vi "search for tag.vi"(8 "error in":errorcluster, 10 "system tag":refnum<class "tag descriptor.lvclass">, 11 "data dictionary in":refnum<class "data dictionary.lvclass">) -> (0 "error out":errorcluster, 2 "index":i32, 3 "data dictionary out":refnum<class "data dictionary.lvclass">)   [LabVIEW 2013, in "tag bus.lvlib" / "data dictionary.lvclass"]
doc: "Uses a tag descriptor to locate a tag within the dictionary. This function uses the name and data type fields of the descriptor."
uses:
  data dictionary.lvclass
  tag/tag descriptor.lvclass
  tag/tag descriptor.lvclass/tag descriptor.ctl
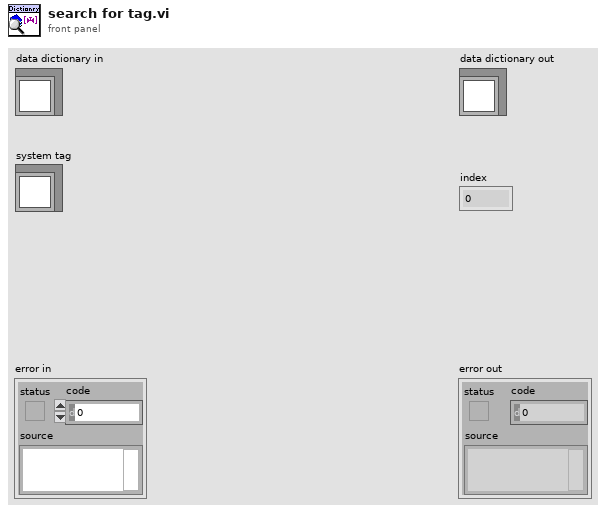
[diagram p1: front panel]
types:
  T1 = typedef "tag bus.lvlib/tag descriptor.lvclass/Data Type.ctl" = enum16{"Double", "Single", "I64", "I32", "I16", "I8", "U64", "U32", "U16", "U8", "Boolean", "String", "Array of Double", "Array of Single", "Array of I64", "Array of I32", "Array of I16", "Array of I8", "Array of U64", "Array of U32", "Array of U16", "Array of U8", "Array of Boolean", "Array of String"}
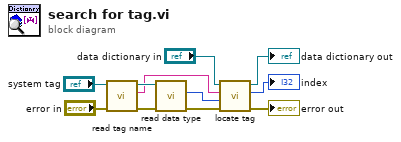
[diagram p0: block diagram]
diagram:
  n1 = call "read tag name.vi"("error in"="error in", "system tag in"="system tag") -> ("error out"=w8:errorcluster, "name"=w4:string, "system tag out"=w10:refnum<class "tag descriptor.lvclass">)  [unwired: 7 in]
  n2 = call "read data type.vi"("error in"=w8, "system tag in"=w10) -> ("error out"=w7:errorcluster, "data type"=w3:T1)  [unwired: 7 in, 1 out]
  n3 = call "locate tag.vi"("error in"=w7, "data type"=w3, "name"=w4, "data dictionary in"="data dictionary in") -> ("error out"=→"error out":errorcluster, "index"=→"index":i32, "data dictionary out"=→"data dictionary out":refnum<class "data dictionary.lvclass">)  [unwired: 5 in]
